vi "BodyBlock.vi"(7 "error in (no error)":errorcluster, 10 "Body":cluster{"Description":string, "Path":path}[](array[cluster])) -> (0 "error out":errorcluster, 2 "Body Out":string, 3 "File Blocks Out":T1(array[cluster]))   [LabVIEW 2016]
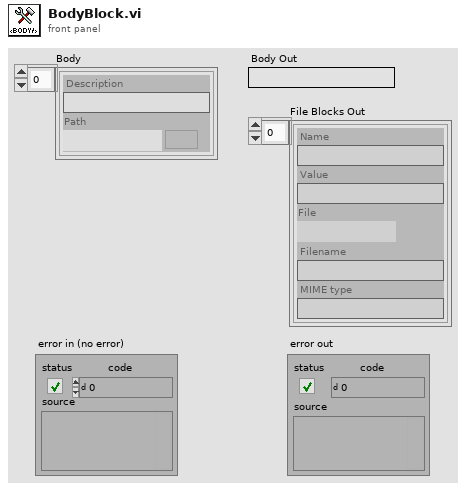
[diagram p1: front panel]
types:
  T1 = cluster{"Name":string, "Value":string, "File":path, "Filename":string, "MIME type":string}[]
  T2 = cluster{"Name":string, "Value":string, "File":path, "Filename":string, "MIME type":string}
  T3 = typedef "imagedata.ctl" = cluster{"image type":i32, "image depth":i32, "image":u8[], "mask":u8[], "colors":u32[], "Rectangle":cluster{"left":i16, "top":i16, "right":i16, "bottom":i16}}
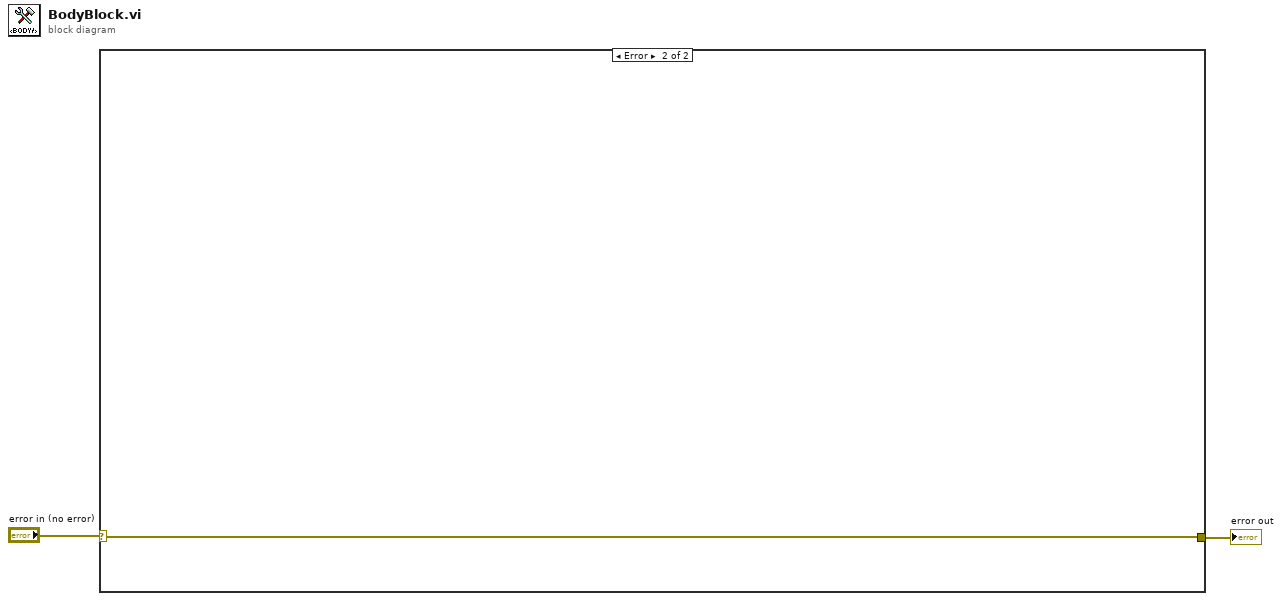
[diagram p0: block diagram]
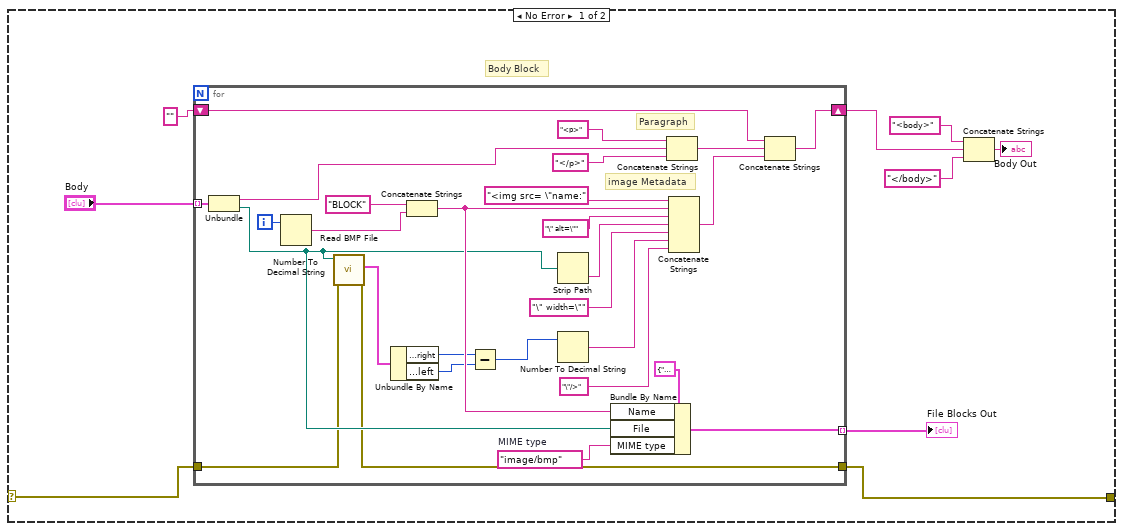
[diagram p2: hidden frame]
diagram:
  n1 = case shown="Error" "error in (no error)" {
    selector: "error in (no error)" -> [w4 w40]
    tunnel: [w3 w40] -> w1
    frame No Error {
      # "Body Block"
      n2 = for {
        tunnel: "Body" -> [w39] mode=indexing
        shift-right: [w17] -> w10
        shift-left: "" -> [w21]
        tunnel: [w33] -> w7 mode=indexing
        tunnel: w4 -> [w13]
        tunnel: [w12] -> w3
        i -> [w37]
        w35 = "image/bmp"  # MIME type
        # "Paragraph"
        # "image Metadata"
        n3 = Unbundle(w39) -> ("Description"=w19:string, "Path"=w16:path)
        n4 = Number To Decimal String(number=w37) -> (decimal integer string=w24:string)  [unwired: 1 in]
        n5 = call <vilib>:"Read BMP File.vi"("error in (no error)"=w13, "path to BMP file"=w16) -> ("error out"=w12:errorcluster, "image data"=w29:T3)  [unwired: 7 in, 1 out]
        n6 = Unbundle By Name(w29) -> ("Rectangle.right"=w15:i16, "Rectangle.left"=w14:i16)
        n7 = Concatenate Strings("BLOCK", w24) -> (w20:string)
        n8 = Subtract(x=w15, y=w14) -> (x-y=w28:i16)
        n9 = Strip Path(path=w16) -> (name=w30:string)  [unwired: 1 out]
        n10 = Number To Decimal String(number=w28) -> (decimal integer string=w26:string)  [unwired: 1 in]
        n11 = Bundle By Name(cluster=T2 {"Name"="", "Value"="", "File"=path "", "Filename"="", "MIME type"="application/octet-stream"} ("Element"), "Name"=w20, "File"=w16, "MIME type"=w35) -> (w33:T2)
        n12 = Concatenate Strings("<p>", w19, "</p>" ("string")) -> (w23:string)
        n13 = Concatenate Strings("<img src= \"name:", w20, "\" alt=\"" ("string"), w30, "\" width=\"" ("string"), w26, "\"/>" ("string")) -> (w22:string)
        n14 = Concatenate Strings(w21, w23, w22) -> (w17:string)
      }
      "File Blocks Out" <- w7
      n15 = Concatenate Strings("<body>" ("string"), w10, "</body>" ("string")) -> (→"Body Out":string)
    }
    frame Error {
    }
  }
  "error out" <- w1
